vi "19_ВПП_Термометр.vi"() -> (0 "Thermometer":dbl(slide) scale=70.0..90.0)   [LabVIEW 2016]
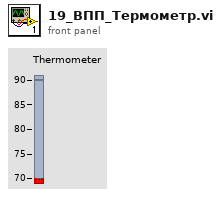
[diagram p1: front panel]
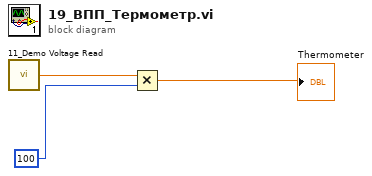
[diagram p0: block diagram]
diagram:
  n1 = call "11_Demo Voltage Read.vi"() -> ("Measured Voltage"=w3:dbl)  [unwired: 2 in]
  n2 = Multiply(x=w3, y=100) -> (x*y=→"Thermometer":dbl)
